vi "Initialize Report.vi"(8 "error in (no error)":errorcluster, 10 "Filepath":path, 11 "Report In":refnum<class "Report.lvclass">) -> (0 "error out":errorcluster, 3 "Report Out":refnum<class "Report.lvclass">)   [LabVIEW 2015, in "Report.lvclass"]
uses:
  Report.lvclass
  Report.lvclass/Report.ctl
  <vilib>/Utility/NIReport.llb/NI_report.lvclass
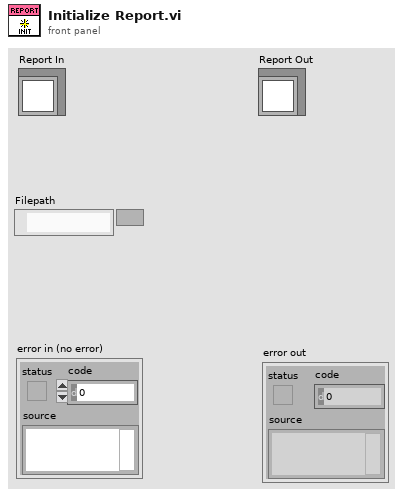
[diagram p1: front panel]
types:
  T1 = enum16{"Standard Report", "HTML", "Word", "Excel"}
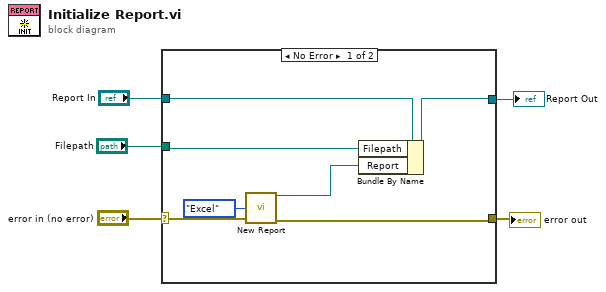
[diagram p0: block diagram]
diagram:
  n1 = case shown="No Error" "error in (no error)" {
    selector: "error in (no error)" -> [w10 w14]
    tunnel: [w7 w14] -> w5
    tunnel: "Report In" -> [w12 w13]
    tunnel: [w11 w13] -> w1
    tunnel: "Filepath" -> [w9 _]
    frame No Error {
      n2 = call <vilib>:"New Report.vi"("report type"=T1."Excel", "error in (no error)"=w10) -> ("report out"=w6:refnum<class "NI_report.lvclass">, "error out"=w7:errorcluster)  [unwired: 12 in]
      n3 = Bundle By Name(cluster=w12, "Filepath"=w9, "Report"=w6) -> (w11:refnum<class "Report.lvclass">)
    }
    frame Error {
    }
  }
  "error out" <- w5
  "Report Out" <- w1
